vi "ByteArray_754IEEEDouble.vi"(3 "Byte Array In":u64, 4 "Output Format":enum16{"IEEE 754 Single", "IEEE 754 Double"}(ring)) -> (5 "IEEE Double Out":dbl)   [LabVIEW 2017, in "Aquisicao de Dados.lvlib"]
uses:
  Aquisicao de Dados.lvlib
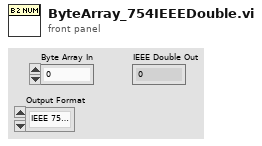
[diagram p1: front panel]
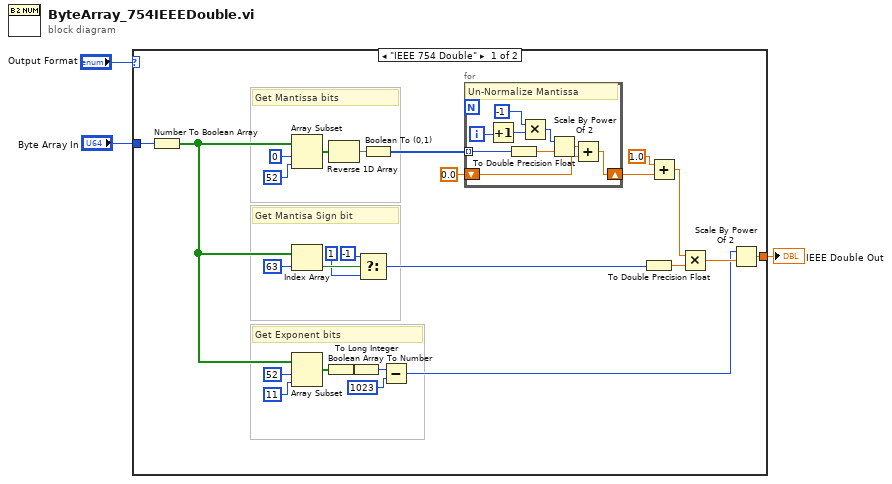
[diagram p0: block diagram]
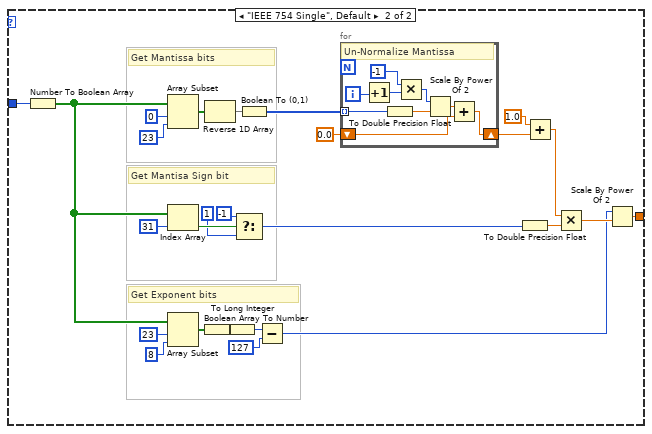
[diagram p2: hidden frame]
diagram:
  n1 = case shown="\"IEEE 754 Double\"" "Output Format" {
    tunnel: [w29 w64] -> w3
    tunnel: "Byte Array In" -> [w27 w62]
    frame "IEEE 754 Double" {
      # "Get Exponent bits"
      # "Get Mantisa Sign bit"
      # "Get Mantissa bits"
      n2 = Number To Boolean Array(number=w27) -> (Boolean array=w28:bool[])
      n3 = Array Subset(array=w28, index=0, length=52) -> (w5:bool[])
      n4 = Index Array(array=w28, index=63) -> (element=w18:bool)
      n5 = Array Subset(array=w28, index=52, length=11) -> (w22:bool[])
      n6 = Boolean Array To Number(Boolean array=w22) -> (number=w21:u32)
      n7 = Reverse 1D Array(array=w5) -> (reversed array=w4:bool[])
      n8 = To Long Integer(number=w21) -> (32bit integer=w15:i32)
      n9 = Select(t=-1 ("index"), s=w18, f=1 ("index")) -> (s? t:f=w10:i32)
      n10 = Boolean To (0,1)(Boolean=w4) -> (0, 1=w14:i16[])
      n11 = Subtract(x=w15, y=1023) -> (x-y=w6:i32)
      n12 = for {
        tunnel: w14 -> [w38] mode=indexing
        shift-right: [w33] -> w12
        shift-left: 0.0 -> [w32]
        i -> [w31]
        # "Un-Normalize Mantissa"
        n13 = Increment(x=w31) -> (x+1=w30:i32)
        n14 = To Double Precision Float(number=w38) -> (double precision float=w37:dbl)
        n15 = Multiply(x=-1, y=w30) -> (x*y=w35:i32)
        n16 = Scale By Power Of 2(n=w35, x=w37) -> (x*2^n=w34:dbl)
        n17 = Add(x=w34, y=w32) -> (x+y=w33:dbl)
      }
      n18 = To Double Precision Float(number=w10) -> (double precision float=w8:dbl)
      n19 = Add(x=1.0, y=w12) -> (x+y=w9:dbl)
      n20 = Multiply(x=w9, y=w8) -> (x*y=w7:dbl)
      n21 = Scale By Power Of 2(n=w6, x=w7) -> (x*2^n=w29:dbl)
    }
    frame "IEEE 754 Single", Default {
      # "Get Exponent bits"
      # "Get Mantisa Sign bit"
      # "Get Mantissa bits"
      n22 = Number To Boolean Array(number=w62) -> (Boolean array=w63:bool[])
      n23 = Array Subset(array=w63, index=0, length=23) -> (w40:bool[])
      n24 = Index Array(array=w63, index=31) -> (element=w53:bool)
      n25 = Array Subset(array=w63, index=23, length=8) -> (w57:bool[])
      n26 = Boolean Array To Number(Boolean array=w57) -> (number=w56:u32)
      n27 = Reverse 1D Array(array=w40) -> (reversed array=w39:bool[])
      n28 = To Long Integer(number=w56) -> (32bit integer=w50:i32)
      n29 = Select(t=-1 ("index"), s=w53, f=1 ("index")) -> (s? t:f=w45:i32)
      n30 = Boolean To (0,1)(Boolean=w39) -> (0, 1=w49:i16[])
      n31 = Subtract(x=w50, y=127) -> (x-y=w41:i32)
      n32 = for {
        tunnel: w49 -> [w73] mode=indexing
        shift-right: [w68] -> w47
        shift-left: 0.0 -> [w67]
        i -> [w66]
        # "Un-Normalize Mantissa"
        n33 = Increment(x=w66) -> (x+1=w65:i32)
        n34 = To Double Precision Float(number=w73) -> (double precision float=w72:dbl)
        n35 = Multiply(x=-1, y=w65) -> (x*y=w70:i32)
        n36 = Scale By Power Of 2(n=w70, x=w72) -> (x*2^n=w69:dbl)
        n37 = Add(x=w69, y=w67) -> (x+y=w68:dbl)
      }
      n38 = To Double Precision Float(number=w45) -> (double precision float=w43:dbl)
      n39 = Add(x=1.0, y=w47) -> (x+y=w44:dbl)
      n40 = Multiply(x=w44, y=w43) -> (x*y=w42:dbl)
      n41 = Scale By Power Of 2(n=w41, x=w42) -> (x*2^n=w64:dbl)
    }
  }
  "IEEE Double Out" <- w3
